vi "CheckDayPassing.vi"(8 "error in":errorcluster, 10 "Data2save.time":dbl[](array[numeric]), 11 "TableName":string) -> (0 "error out":errorcluster, 1 "split-index":i32, 2 "Split array":bool, 4 "TimeValid":bool, 5 "DayName2":string, 7 "DayName1":string)   [LabVIEW 2020, in "DBAL-BIN.lvclass"]
doc: "This VI will check if the time of the dataset is passing one day.\nIf that is the case, then the dataset has to be split in two subsections and processed separately."
uses:
  DBAL-BIN.lvclass
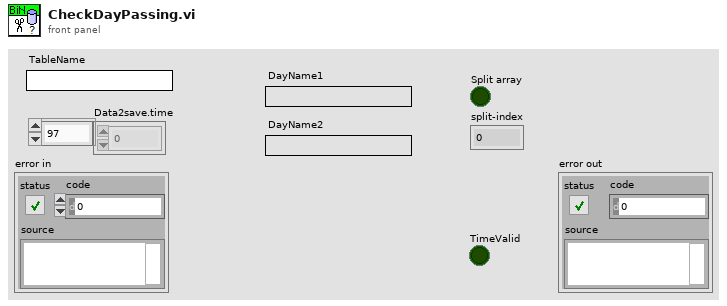
[diagram p1: front panel]
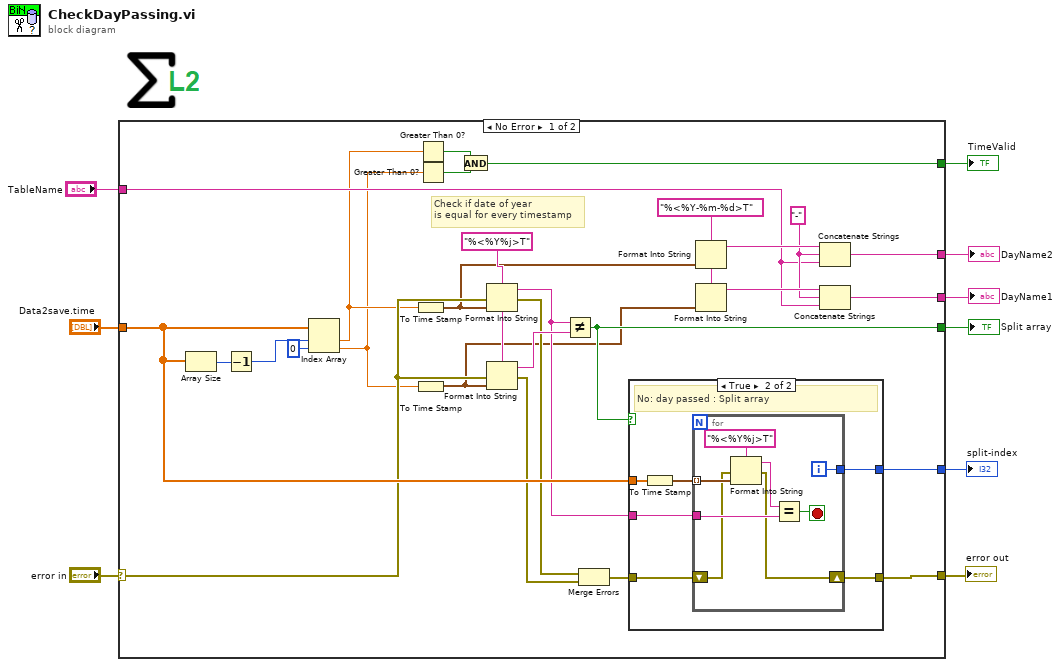
[diagram p0: block diagram]
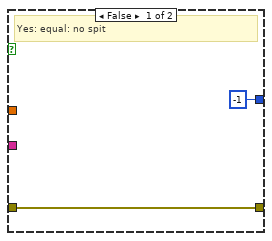
[diagram p2: hidden frame]
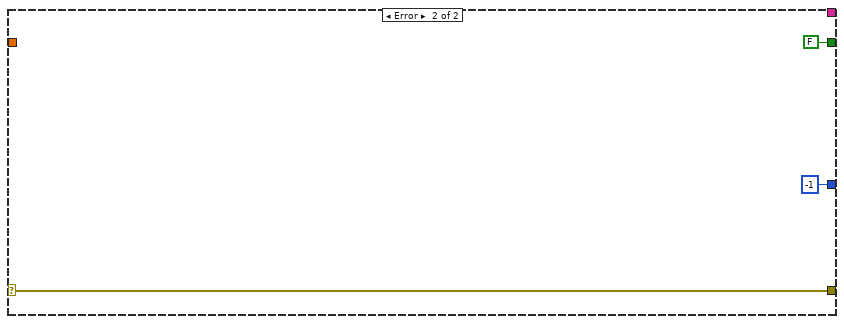
[diagram p3: hidden frame]
diagram:
  n1 = case shown="No Error" "error in" {
    selector: "error in" -> [w25 w56]
    tunnel: "Data2save.time" -> [w33 _]
    tunnel: [w31 -1] -> w8
    tunnel: [w26 w56] -> w7
    tunnel: [w24 FALSE] -> w5
    tunnel: [w16 _] -> w4
    tunnel: [w15 _] -> w3
    tunnel: "TableName" -> [w17 _]
    tunnel: [w10 _] -> w1
    frame No Error {
      w18 = "-" ("initial string")
      w21 = "%<%Y-%m-%d>T" ("format string")
      w34 = "%<%Y%j>T" ("format string")
      # "Check if date of year\nis equal for every timestamp"
      n2 = Array Size(array=w33) -> (size(s)=w37:i32)
      n3 = Decrement(x=w37) -> (x-1=w36:i32)
      n4 = Index Array(array=w33, index #1=w36, index #2=0 ("index")) -> (element #1=w14:dbl, element #2=w13:dbl)
      n5 = To Time Stamp(1:w14) -> (0:w22:timestamp)
      n6 = To Time Stamp(1:w13) -> (0:w23:timestamp)
      n7 = Greater Than 0?(x=w14) -> (x > 0?=w12:bool)
      n8 = Greater Than 0?(x=w13) -> (x > 0?=w11:bool)
      n9 = And(x=w12, y=w11) -> (x .and. y?=w10:bool)
      n10 = Format Into String(format string=w34, error in=w25, w22) -> (resulting string=w30:string, error out=w29:errorcluster)  [unwired: 1 in]
      n11 = Format Into String(format string=w34, error in=w25, w23) -> (resulting string=w32:string, error out=w28:errorcluster)  [unwired: 1 in]
      n12 = Not Equal?(x=w30, y=w32) -> (x != y?=w24:bool)
      n13 = Merge Errors(w29, w28) -> (w27:errorcluster)
      n14 = case shown="True" w24 {
        tunnel: w33 -> [_ w45]
        tunnel: w30 -> [_ w43]
        tunnel: [-1 w42] -> w31
        tunnel: w27 -> [w38 w41]
        tunnel: [w38 w40] -> w26
        frame False {
          # "Yes: equal: no spit"
        }
        frame True {
          # "No: day passed : Split array"
          n15 = To Time Stamp(1:w45) -> (0:w44:timestamp[])
          n16 = for {
            tunnel: w44 -> [w52] mode=indexing
            tunnel: w43 -> [w50]
            tunnel: [w48] -> w42
            shift-right: [w46] -> w40
            shift-left: w41 -> [w47]
            i -> [w48]
            stop <- w49 stop-if-true
            n17 = Format Into String(format string="%<%Y%j>T", error in=w47, w52) -> (resulting string=w51:string, error out=w46:errorcluster)  [unwired: 1 in]
            n18 = Equal?(x=w51, y=w50) -> (x = y?=w49:bool)
          }
        }
      }
      n19 = Format Into String(format string=w21, w22) -> (resulting string=w20:string)  [unwired: 2 in, 1 out]
      n20 = Format Into String(format string=w21, w23) -> (resulting string=w19:string)  [unwired: 2 in, 1 out]
      n21 = Concatenate Strings(w20, w18, w17) -> (w16:string)
      n22 = Concatenate Strings(w19, w18, w17) -> (w15:string)
    }
    frame Error {
    }
  }
  "split-index" <- w8
  "error out" <- w7
  "Split array" <- w5
  "DayName1" <- w3
  "DayName2" <- w4
  "TimeValid" <- w1
